vi "XC_fits.vi"(4 "Cursor Position1":dbl, 5 "Cursor Position0":dbl, 6 "Background":bool, 7 "Filter":bool, 8 "initial parameters":dbl[](array[numeric]), 9 "?":enum16{"Lorantzian", "fano", "gaussian"}(ring)=enum."gaussian", 10 "parameter bounds":T1={"amp min"=-inf, "amp max"=inf, "deviation min"=-inf, "deviation max"=inf, "offset min"=0.0, "offset max"=0.0}, 11 "file path (dialog if empty)":path) -> (2 "Intensity Graph":dbl[][](graph), 3 "Waveform Graph":dynamicdata(graph))   [LabVIEW 2014]
uses:
  <vilib>/Utility/file.llb/Read From Spreadsheet File (DBL).vi
  <vilib>/Analysis/Matrix/Numeric/Conversions/Array To Matrix - RA2.vi
  <vilib>/Math Plots/3D Math Plots/3D Surface/3D Surface Datatype/Public/Plot Helper (Vector).vi
  <vilib>/Analysis/Matrix/NI_Matrix.lvlib
  <vilib>/Math Plots/3D Math Plots/3D Surface/3D Surface Datatype/3D Surface Datatype.lvclass
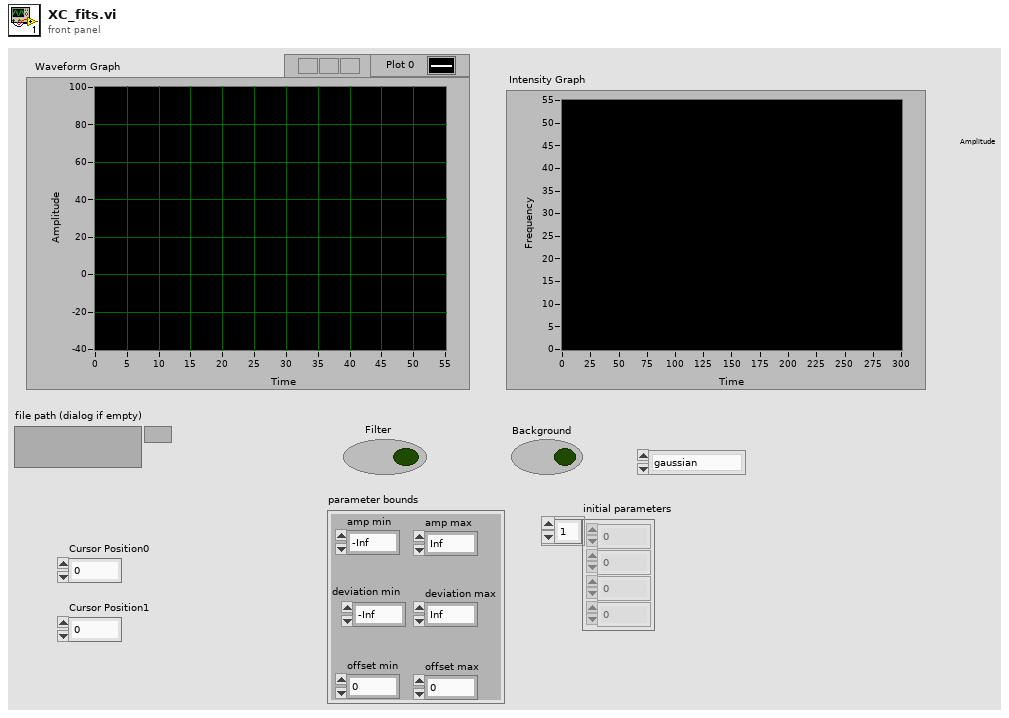
[diagram p1: front panel]
types:
  T1 = cluster{"amp min":dbl, "amp max":dbl, "deviation min":dbl, "deviation max":dbl, "offset min":dbl, "offset max":dbl}
  T2 = cluster{"amp min":dbl, "amp max":dbl, dbl, dbl, "deviation min":dbl, "deviation max":dbl, "offset min":dbl, "offset max":dbl}
  T3 = cluster{dbl, "result":dbl, dbl, "delta amplitude":dbl, dbl, "delta standard deviation":dbl, "center":dbl, "delta center":dbl}
  T4 = typedef "NI_Matrix.lvlib/RealMatrix.ctl" = dbl[][]
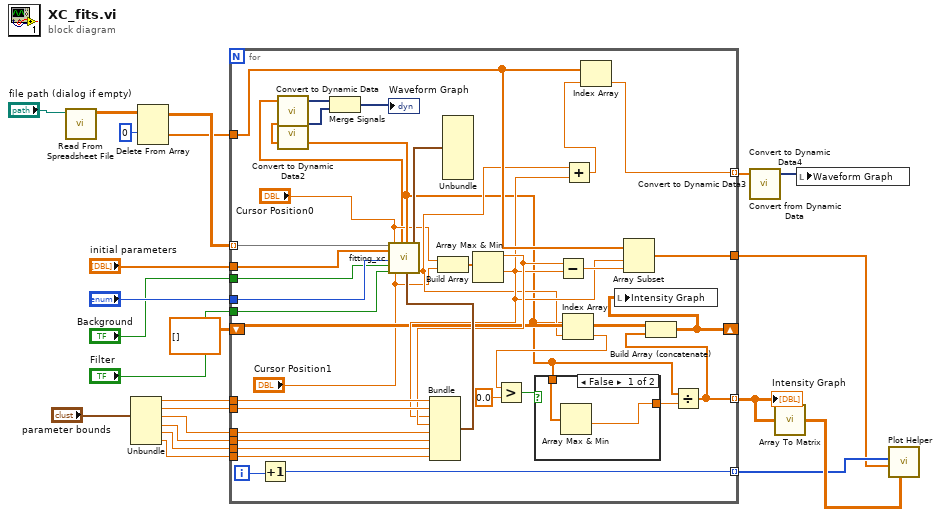
[diagram p0: block diagram]
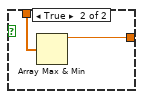
[diagram p2: hidden frame]
diagram:
  n1 = call-poly <vilib>:"Read From Spreadsheet File.vi"("file path (dialog if empty)"="file path (dialog if empty)") -> ("all rows"=w25:dbl[][])  [unwired: 6 in, 4 out]
  n2 = Unbundle("parameter bounds") -> ("amp min"=w17:dbl, "amp max"=w16:dbl, "deviation min"=w15:dbl, "deviation max"=w14:dbl, "offset min"=w13:dbl, "offset max"=w12:dbl)
  n3 = Delete From Array(array=w25, index (row)=0) -> (deleted portion=w9:dbl[], array with subset deleted=w23:dbl[][])  [unwired: 2 in]
  n4 = for {
    tunnel: w23 -> [w48] mode=indexing
    tunnel: "initial parameters" -> [w63]
    tunnel: "?" -> [w62]
    tunnel: "Background" -> [w61]
    tunnel: "Filter" -> [w60]
    tunnel: w17 -> [w59]
    tunnel: w16 -> [w58]
    tunnel: w15 -> [w57]
    tunnel: w14 -> [w56]
    tunnel: w13 -> [w55]
    tunnel: w12 -> [w54]
    tunnel: [w49] -> w11 mode=indexing
    tunnel: w9 -> [w44]
    tunnel: [w31] -> w4 mode=indexing
    tunnel: [w43] -> w3
    tunnel: [w30] -> w6 mode=indexing
    shift-right: [w34] -> _
    shift-left: dbl[][] [] -> [w33]
    i -> [w35]
    n5 = Increment(x=w35) -> (x+1=w31:i32)
    n6 = Build Array("Cursor Position0", "Cursor Position1") -> (w53:dbl[])
    n7 = Array Max & Min(array=w53) -> (max value=w42:dbl, min value=w41:dbl)  [unwired: 2 out]
    n8 = Bundle("amp min"=w59, "amp max"=w58, w41, w42, "deviation min"=w57, "deviation max"=w56, "offset min"=w55, "offset max"=w54) -> (w52:T2)  [unwired: 1 in]
    n9 = call "fitting_xc.vi"("array"=w48, "initial parameters"=w63, "Enum"=w62, "Background"=w61, "Filter"=w60, "x"="Cursor Position0", "x 2"="Cursor Position1", "parameter bounds"=w52) -> ("sub_Y"=w27:dbl[], "Best Gaussian Fit"=w29:dbl[], "output cluster"=w51:T3, "center"=w32:dbl)  [unwired: 6 in, 2 out]
    n10 = call "Convert to Dynamic Data"("Array"=w27) -> ("Dynamic Data Type"=w47:dynamicdata)  [unwired: 3 in]
    n11 = call "Convert to Dynamic Data2"("Array"=w29) -> ("Dynamic Data Type"=w46:dynamicdata)  [unwired: 3 in]
    n12 = Merge Signals(w47, w46) -> (→"Waveform Graph":dynamicdata)
    n13 = Unbundle(w51) -> ()  [unwired: 8 out]
    n14 = Subtract(x=w42, y=w41) -> (x-y=w45:dbl)
    n15 = Index Array(array=w29, index=w32) -> (element=w38:dbl)
    n16 = Greater?(x=w38, y=0.0) -> (0:w37:bool)
    n17 = case shown="False" w37 {
      tunnel: w29 -> [w64 w67]
      tunnel: [w65 w66] -> w36
      frame False {
        n18 = Array Max & Min(array=w64) -> (min value=w65:dbl)  [unwired: 3 out]
      }
      frame True {
        n19 = Array Max & Min(array=w67) -> (max value=w66:dbl)  [unwired: 3 out]
      }
    }
    n20 = Add(x=w32, y=w41) -> (x+y=w50:dbl)
    n21 = Index Array(array=w44, index=w50) -> (element=w49:dbl)
    n22 = Array Subset(array=w44, index=w41, length=w45) -> (w43:dbl[])
    n23 = Divide(x=w29, y=w36) -> (x/y=w30:dbl[])
    n24 = Build Array (concatenate)(w33, w30) -> (w34:dbl[][])
    n25 = local write "Intensity Graph"(w34) -> ()
  }
  "Intensity Graph" <- w6
  n26 = call "Convert to Dynamic Data3"("Array"=w11) -> ("Dynamic Data Type"=w10:dynamicdata)  [unwired: 3 in]
  n27 = call "Convert from Dynamic Data"("Dynamic Data Type"=w10) -> ("Array"=w8:dbl[])  [unwired: 3 in]
  n28 = call "Convert to Dynamic Data4"("Array"=w8) -> ("Dynamic Data Type"=w7:dynamicdata)  [unwired: 3 in]
  n29 = call-poly <vilib>:"Array To Matrix.vi"("Real 2D Array"=w6) -> ("Real Matrix"=w5:T4)
  n30 = local write "Waveform Graph"(w7) -> ()
  n31 = call-poly <vilib>:"Plot Helper.vi"("z matrix"=w5, "y vector"=w3, "x vector"=w4) -> ()  [unwired: 3 in, 6 out]
